vi "ni_move_backlash.vi"(6 "Axis enable":bool[](array[boolean])=[TRUE, TRUE, TRUE, TRUE], 8 "error in":errorcluster, 9 "Axis positions":dbl[](array[numeric]), 10 "Absolute":bool=TRUE) -> (0 "error out":errorcluster, 1 "Final axis errors":i32[](array[numeric]))   [LabVIEW 2014]
panel:
  out "Pull-in errors":i32[][](graph)
  out "Pull in iterations":i32
  in  "Pull in gain":dbl=0.8
  in  "Clear histogram":bool
  in  "Histogram N":i32=10
  out "Error histogram":cluster{"X":i32[], "Y":i32[]}[](graph)
  in  "Pull in offset":i32=15
  in  "Backlash offset":i32=100
  # "Diagnostics"
  # "The controller axis numbers (starting from 1)"
  # "Like ni_move.vi, but always approaches the position in the + direction.  This minimizes the contribution of backlash to nonrepeatability.  For this to work, pull-in moves must be set to 0 for the axes so that the motion controller won't try to back up."
  # "Parameters:"
  # "Amount we offset position by when approaching from the reverse direction.  Some value greater than the backlash (in steps.)"
  # "Amount we stop short in direction of travel.  Some value (in steps) more than the typical open-loop error, but well less than a full step.  This way our pull-in move is always in the right direction."
  # "Fraction of remaining distance we pull in on each move."
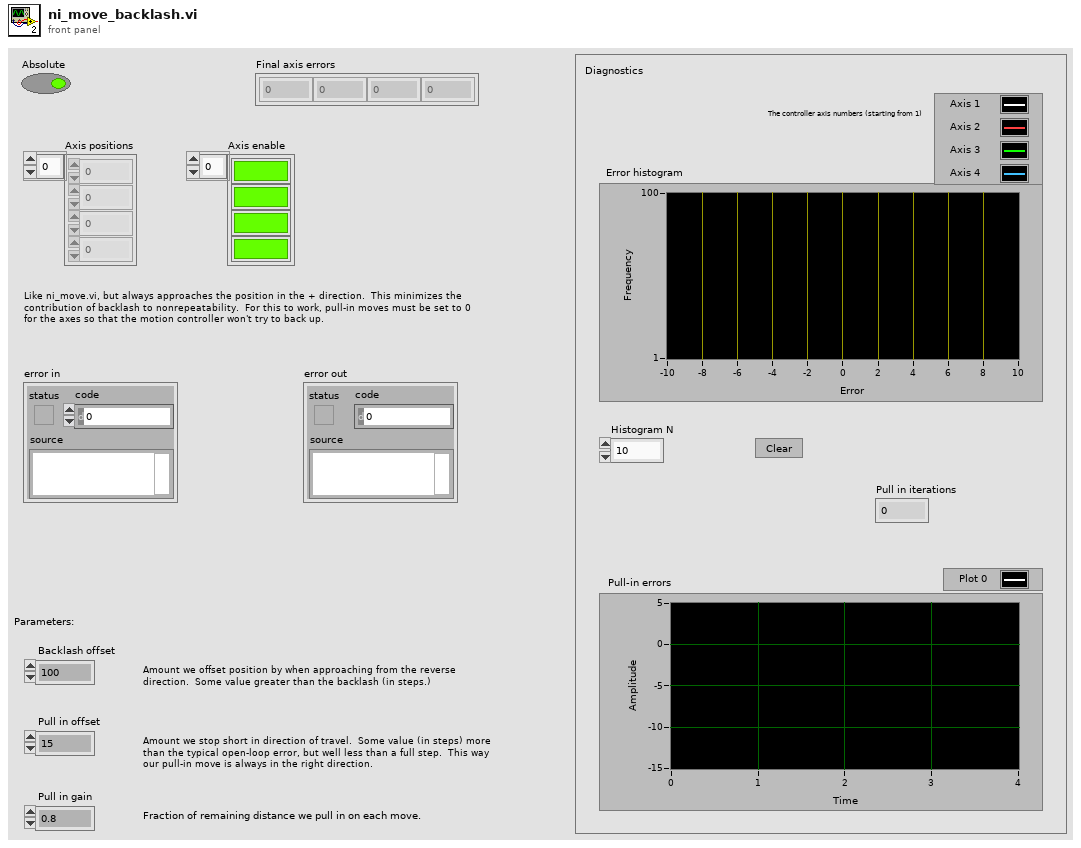
[diagram p1: front panel]
types:
  T1 = typedef "Board Id" = u8
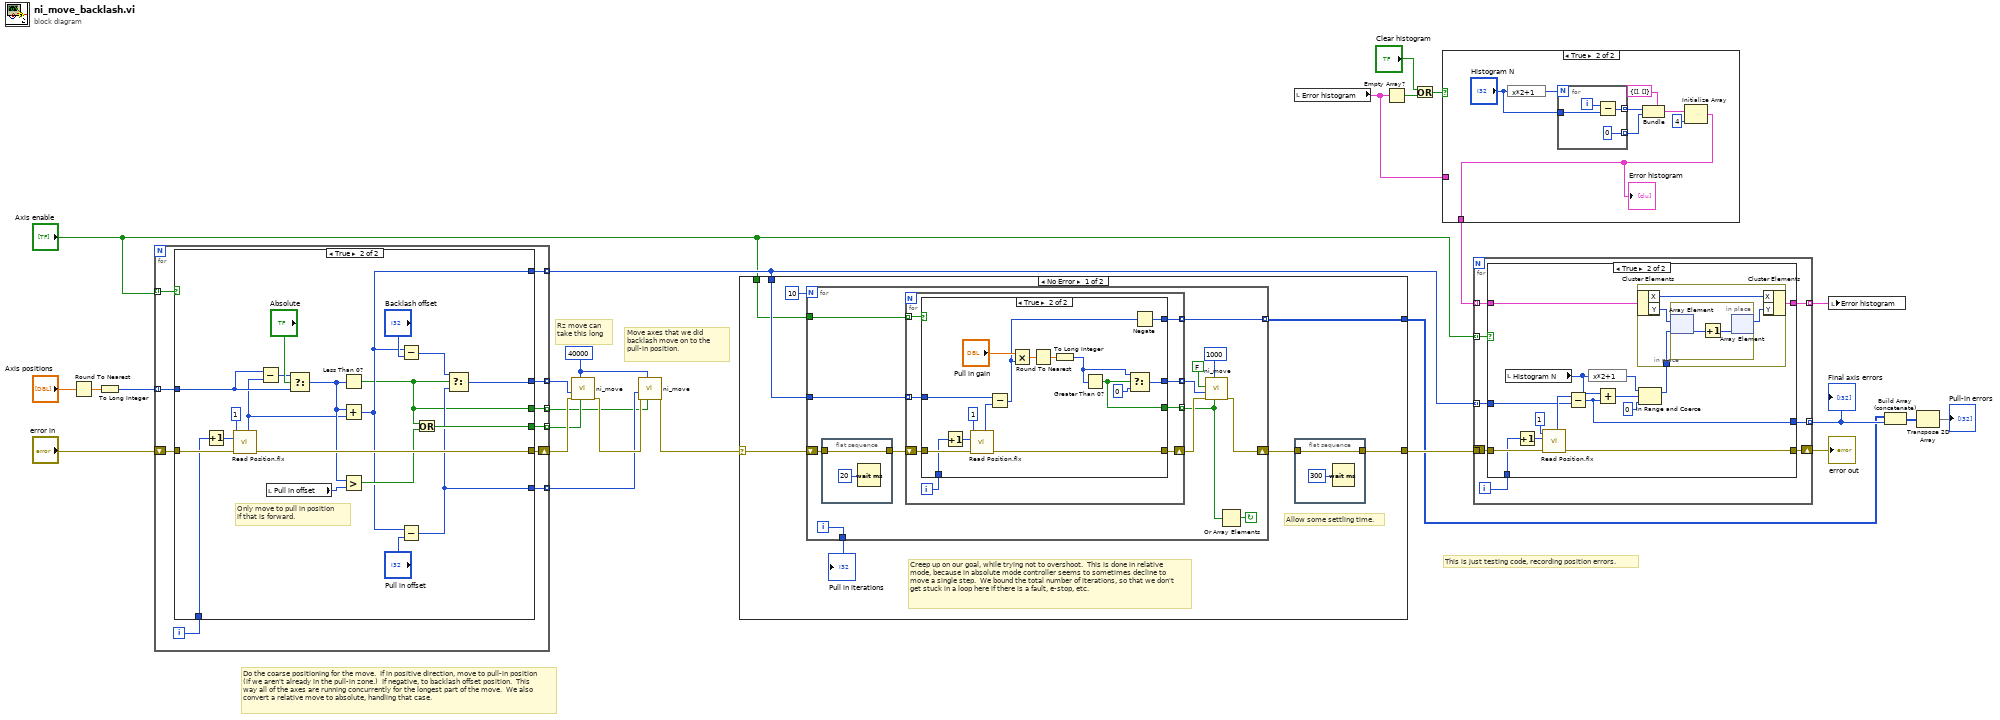
[diagram p0: block diagram]
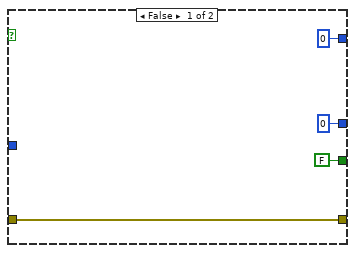
[diagram p2: hidden frame]
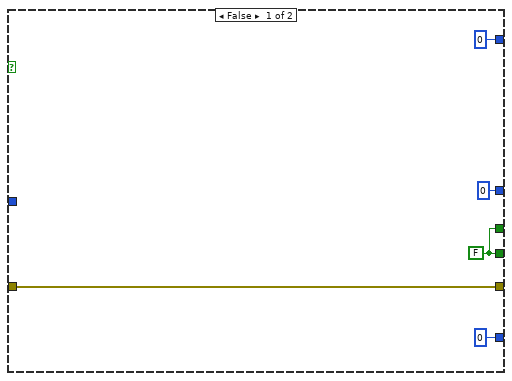
[diagram p4: hidden frame]
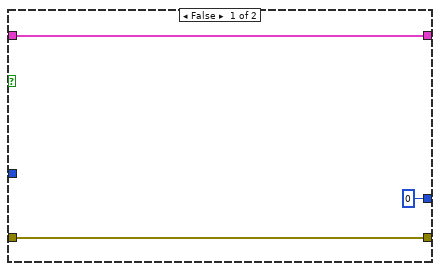
[diagram p6: hidden frame]
diagram:
  w1 = u32 40000 ("Timeout")
  # "Rz move can take this long"
  # "Move axes that we did backlash move on to the pull-in position."
  # "Do the coarse positioning for the move.  If in positive direction, move to pull-in position (if we aren't already in the pull-in zone.)  If negative, to backlash offset position.  This way all of the axes are running concurrently for the longest part of the move.  We also convert a relative move to absolute, handling that case."
  # "This is just testing code, recording position errors."
  n1 = Round To Nearest(number="Axis positions") -> (nearest integer value=w25:dbl[])
  n2 = To Long Integer(number=w25) -> (32bit integer=w23:i32[])
  n3 = for {
    tunnel: "Axis enable" -> [w35] mode=indexing
    tunnel: w23 -> [w34] mode=indexing
    shift-right: [w33] -> w7
    shift-left: "error in" -> [w36]
    tunnel: [w31] -> w5 mode=indexing
    tunnel: [w30] -> w22 mode=indexing
    tunnel: [w29] -> w8 mode=indexing
    tunnel: [w28] -> w4 mode=indexing
    tunnel: [w27] -> w3 mode=indexing
    i -> [w32]
    n4 = case shown="True" w35 {
      tunnel: w36 -> [w41 w60]
      tunnel: w32 -> [_ w55]
      tunnel: w34 -> [_ w57]
      tunnel: [w41 w56] -> w33
      tunnel: [w38 w49] -> w31
      tunnel: [0 w46] -> w30
      tunnel: [0 w44] -> w29
      tunnel: [0 w43] -> w28
      tunnel: [w38 w42] -> w27
      frame False {
        w38 = FALSE
      }
      frame True {
        # "Only move to pull in position\nif that is forward."
        n5 = Increment(x=w55) -> (x+1=w54:i32)
        n6 = call <vilib>:"Read Position.flx"("error in (no error)"=w60, "Axis"=w54, "Board ID"=T1 1) -> ("error out"=w56:errorcluster, "Position"=w47:i32)  [unwired: 3 in, 2 out]
        n7 = Subtract(x=w57, y=w47) -> (x-y=w58:i32)
        n8 = local read "Pull in offset"() -> (w52:i32)
        n9 = Select(t=w58, s="Absolute", f=w57) -> (s? t:f=w50:i32)
        n10 = Less Than 0?(x=w50) -> (x < 0?=w42:bool)
        n11 = Add(x=w50, y=w47) -> (x+y=w46:i32)
        n12 = Greater?(x=w50, y=w52) -> (0:w51:bool)
        n13 = Subtract(x=w46, y="Backlash offset") -> (x-y=w45:i32)
        n14 = Subtract(x=w46, y="Pull in offset") -> (x-y=w43:i32)
        n15 = Or(x=w42, y=w51) -> (x .or. y?=w49:bool)
        n16 = Select(t=w45, s=w42, f=w43) -> (s? t:f=w44:i32)
      }
    }
  }
  n17 = call "ni_move.vi"("Axis enable"=w5, "Timeout"=w1, "error in"=w7, "Axis positions"=w8) -> ("error out"=w6:errorcluster)  [unwired: 7 in]
  n18 = call "ni_move.vi"("Axis enable"=w3, "Timeout"=w1, "error in"=w6, "Axis positions"=w4) -> ("error out"=w2:errorcluster)  [unwired: 7 in]
  n19 = case shown="No Error" w2 {
    selector: w2 -> [w64 w115]
    tunnel: w22 -> [w69 _]
    tunnel: [w63 w115] -> w18
    tunnel: [w66 _] -> w10
    tunnel: "Axis enable" -> [w65 _]
    frame No Error {
      # "Allow some settling time."
      # "Creep up on our goal, while trying not to overshoot.  This is done in relative mode, because in absolute mode controller seems to sometimes decline to move a single step.  We bound the total number of iterations, so that we don't get stuck in a loop here if there is a fault, e-stop, etc."
      n20 = for {
        N: 10 -> [_]
        tunnel: w65 -> [w82]
        tunnel: w69 -> [w81]
        tunnel: [w78] -> w68
        tunnel: [w73] -> w66 mode=indexing
        shift-right: [w80] -> w62
        shift-left: w64 -> [w75]
        i -> [w78]
        stop <- w77 continue-if-true
        n21 = flat-sequence {
          tunnel: w75 -> [w85]
          tunnel: [w85] -> w74
          frame #0 {
            n22 = Wait (ms)(milliseconds to wait=u32 20) -> ()  [unwired: 1 out]
          }
        }
        n23 = for {
          tunnel: w82 -> [w93] mode=indexing
          tunnel: w81 -> [w92] mode=indexing
          shift-right: [w91] -> w84
          shift-left: w74 -> [w94]
          tunnel: [w89] -> w79 mode=indexing
          tunnel: [w88] -> w83 mode=indexing
          tunnel: [w87] -> w73 mode=indexing
          i -> [w90]
          n24 = case shown="True" w93 {
            tunnel: w94 -> [w98 w112]
            tunnel: w90 -> [_ w108]
            tunnel: w92 -> [_ w106]
            tunnel: [w98 w111] -> w91
            tunnel: [FALSE w114] -> w89
            tunnel: [0 w110] -> w88
            tunnel: [0 w99] -> w87
            frame False {
            }
            frame True {
              n25 = Increment(x=w108) -> (x+1=w107:i32)
              n26 = call <vilib>:"Read Position.flx"("error in (no error)"=w112, "Axis"=w107, "Board ID"=T1 1) -> ("error out"=w111:errorcluster, "Position"=w104:i32)  [unwired: 3 in, 2 out]
              n27 = Subtract(x=w106, y=w104) -> (x-y=w100:i32)
              n28 = Multiply(x="Pull in gain", y=w100) -> (x*y=w103:dbl)
              n29 = Round To Nearest(number=w103) -> (nearest integer value=w102:dbl)
              n30 = To Long Integer(number=w102) -> (32bit integer=w101:i32)
              n31 = Greater Than 0?(x=w101) -> (x > 0?=w114:bool)
              n32 = Select(t=w101, s=w114, f=0) -> (s? t:f=w110:i32)
              n33 = Negate(x=w100) -> (-x=w99:i32)
            }
          }
        }
        n34 = call "ni_move.vi"("Axis enable"=w79, "Timeout"=u32 1000, "error in"=w84, "Axis positions"=w83, "Absolute"=FALSE) -> ("error out"=w80:errorcluster)  [unwired: 6 in]
        n35 = Or Array Elements(Boolean array=w79) -> (logical OR=w77:bool)
      }
      "Pull in iterations" <- w68
      n36 = flat-sequence {
        tunnel: [w70] -> w63
        tunnel: w62 -> [w70]
        frame #0 {
          n37 = Wait (ms)(milliseconds to wait=u32 300) -> ()  [unwired: 1 out]
        }
      }
    }
    frame Error {
    }
  }
  n38 = local read "Error histogram"() -> (w21:cluster{"X":i32[], "Y":i32[]}[])
  n39 = Empty Array?(array=w21) -> (empty?=w16:bool)
  n40 = Or(x="Clear histogram", y=w16) -> (x .or. y?=w15:bool)
  n41 = case shown="True" w15 {
    tunnel: w21 -> [w116 _]
    tunnel: [w116 w117] -> w20
    frame False {
      # "Histogram initialized"
    }
    frame True {
      n42 = expression code="x*2+1"("Histogram N") -> (w124:i32)
      n43 = for {
        N: w124 -> [_]
        tunnel: "Histogram N" -> [w127]
        tunnel: [w126] -> w122 mode=indexing
        tunnel: [0 ("Histogram N")] -> w121 mode=indexing
        i -> [w128]
        n44 = Subtract(x=w128, y=w127) -> (x-y=w126:i32)
      }
      n45 = Bundle(cluster=cluster{"X":i32[], "Y":i32[]} {"X"=[], "Y"=[]}, "X"=w122, "Y"=w121) -> (w120:cluster{"X":i32[], "Y":i32[]})
      n46 = Initialize Array(w120, 4 ("dimension size")) -> (w117:cluster{"X":i32[], "Y":i32[]}[])
      "Error histogram" <- w117
    }
  }
  n47 = for {
    tunnel: "Axis enable" -> [w135] mode=indexing
    tunnel: w22 -> [w134] mode=indexing
    shift-right: [w133] -> w19
    shift-left: _ -> [w136]
    tunnel: w20 -> [w131] mode=indexing
    tunnel: [w130] -> w14 mode=indexing
    tunnel: w18 -> [_]
    tunnel: [w129] -> w13 mode=indexing
    i -> [w132]
    n48 = case shown="True" w135 {
      tunnel: w136 -> [w139 w153]
      tunnel: w132 -> [_ w145]
      tunnel: w134 -> [_ w143]
      tunnel: [w139 w152] -> w133
      tunnel: w131 -> [w138 w149]
      tunnel: [w138 w147] -> w130
      tunnel: [0 w142] -> w129
      frame False {
      }
      frame True {
        n49 = local read "Histogram N"() -> (w141:i32)
        n50 = Increment(x=w145) -> (x+1=w146:i32)
        n51 = call <vilib>:"Read Position.flx"("error in (no error)"=w153, "Axis"=w146, "Board ID"=T1 1) -> ("error out"=w152:errorcluster, "Position"=w144:i32)  [unwired: 3 in, 2 out]
        n52 = Subtract(x=w144, y=w143) -> (x-y=w142:i32)
        n53 = expression code="x*2+1"(w141) -> (w140:i32)
        n54 = Add(x=w141, y=w142) -> (x+y=w151:i32)
        n55 = In Range and Coerce(upper limit=w140, x=w151, lower limit=0) -> (coerced(x)=w148:i32)  [unwired: 1 out]
        n56 = in-place {
          in-place-border: w148 -> [w156]
          n57 = in-place-cluster #1(w149) -> ("X"=w158:i32[], "Y"=w157:i32[])
          n58 = in-place {
            n59 = in-place-array #2(w157, w156) -> (w160:i32)
            n60 = Increment(x=w160) -> (x+1=w159:i32)
            n61 = in-place-array #2(w159) -> (w155:i32[])  [unwired: 1 out]
          }
          n62 = in-place-cluster #1("X"=w158, "Y"=w155) -> (w147:cluster{"X":i32[], "Y":i32[]})
        }
      }
    }
  }
  "error out" <- w19
  "Final axis errors" <- w13
  n63 = local write "Error histogram"(w14) -> ()
  n64 = Build Array (concatenate)(w10, w13) -> (w12:i32[][])
  n65 = Transpose 2D Array(2D array=w12) -> (transposed array=→"Pull-in errors":i32[][])
